vi "Yahoo - URL - Build (for stock ticker).vi"(0 "Symbol":string, 3 "error in":errorcluster) -> (6 "URL (Pre-redirect)":string, 7 "URL (Post-redirect)":string, 9 "error out":errorcluster)   [LabVIEW 2011]
doc: "Build the URL required to retrieve the stock data from Yahoo Finance.\nTwo URLs are necessary as the first one results in a redirect 130 with new URL.\nThis new URL is predictable from the first one so it is generated in advance.\n\nInputs:\n Symbol: Stock ticker symbol.\n Error in: Describes error conditions that occur before this node runs. This input provides standard error in functionality.\n\nOutputs:\n URL (Pre-redirect): URL of the first HTTP request.\n URL (Post-redirect): URL of the second HTTP request.\n Error out: Contains error information. This output provides standard error out functionality."
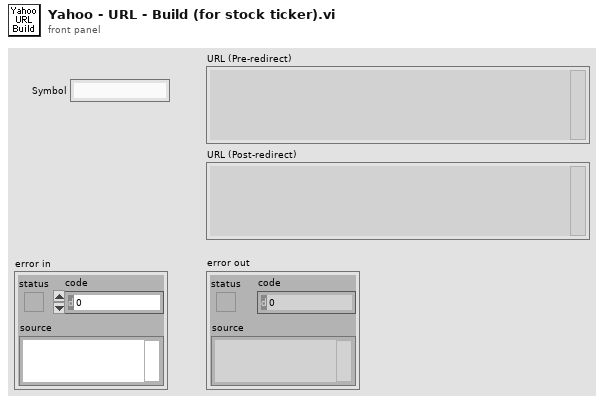
[diagram p1: front panel]
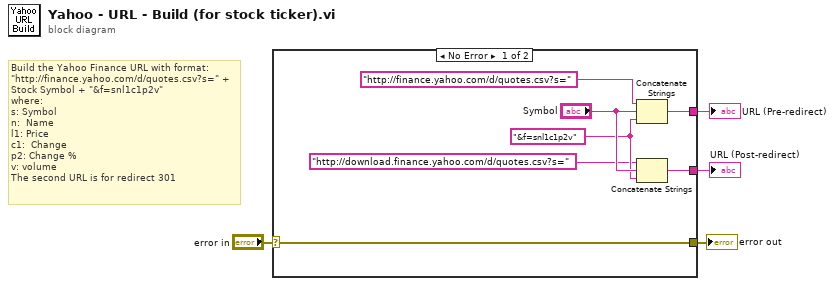
[diagram p0: block diagram]
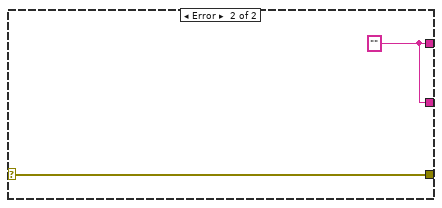
[diagram p2: hidden frame]
diagram:
  # "Build the Yahoo Finance URL with format:\n\"http://finance.yahoo.com/d/quotes.csv?s=\" +\nStock Symbol + \"&f=snl1c1p2v\"\nwhere:\ns: Symbol\nn:  Name\nl1: Price\nc1:  Change\np2: Change %\nv: volume\nThe second URL is for redirect 301"
  n1 = case shown="No Error" "error in" {
    selector: "error in" -> [w9 w13]
    tunnel: [w10 w12] -> w4
    tunnel: [w9 w13] -> w3
    tunnel: [w5 w12] -> w1
    frame No Error {
      w7 = "&f=snl1c1p2v" ("string")
      n2 = Concatenate Strings("http://finance.yahoo.com/d/quotes.csv?s=" ("string"), "Symbol", w7) -> (w10:string)
      n3 = Concatenate Strings("http://download.finance.yahoo.com/d/quotes.csv?s=" ("string"), "Symbol", w7) -> (w5:string)
    }
    frame Error {
      w12 = ""
    }
  }
  "URL (Pre-redirect)" <- w4
  "error out" <- w3
  "URL (Post-redirect)" <- w1
